vi "总磷氨氮插入数据.vi"(0 "database":string, 1 "data":T2 {"单位" items=["ug/L", "mg/L", "ppm", "mg/m3", "cm", "ppb", "ug/m3", "%", "nmol/mol", "umol/mol", "MPN/L", "MPN/100ml", "ng/m3", "NTU", "无量纲", "ms/cm", "us/cm"]}, 3 "SN":string, 5 "table":string, 7 "测量模式":T1(ring)=enum."水样测试", 9 "数据标记表":string(combo)="N", 11 "error in (no error)":errorcluster) -> (15 "error out":errorcluster)   [LabVIEW 2016, in "database.lvlib"]
uses:
  database.lvlib
  <vilib>/Utility/sysdir.llb/System Directory Type.ctl
  <vilib>/addons/database/Connection.llb/DB Tools Open Connec (String).vi
  <vilib>/addons/database/Connection.llb/Conn Execute.vi
  <vilib>/addons/database/Recordset.llb/Rec Fetch Recordset Data (R).vi
  <vilib>/addons/database/Recordset.llb/Rec Destroy - Connection.vi
  <vilib>/addons/database/NI_Database_API.lvlib
panel:
  out "为空？":bool
  out "recordset data":variant[][](array[variant])
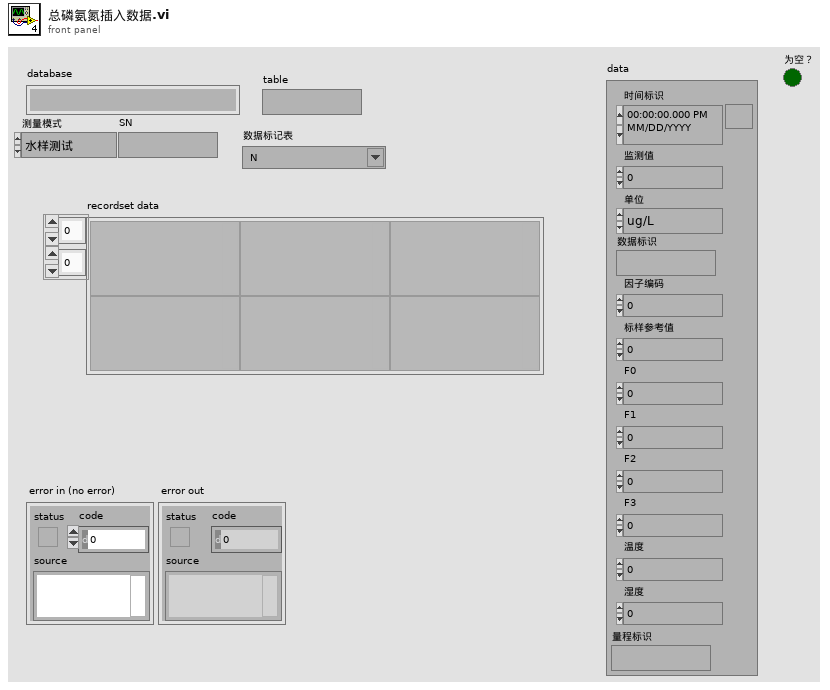
[diagram p1: front panel]
types:
  T1 = enum16{"维护数据", "水样测试", "标样核查", "零点核查", "跨度核查", "空白测试", "平行样测试", "加标回收", "空白校准", "标样校准", "初始化（清洗）"}
  T2 = cluster{"时间标识":timestamp, "监测值":sgl, "单位":u16, "数据标识":string, "因子编码":u32, "标样参考值":sgl, "F0":sgl, "F1":sgl, "F2":sgl, "F3":sgl, "温度":sgl, "湿度":sgl, "量程标识":string}
  T3 = typedef "System Directory Type.ctl" = i32
  T4 = typedef "NI_Database_API.lvlib/Conn ObjectReference.ctl" = refnum<k1>
  T5 = typedef "NI_Database_API.lvlib/Rec ObjectReference.ctl" = refnum<k1>
  T6 = cluster{"时间标识":timestamp, "测量模式":string, "数据类型":string, "监测值":sgl, "单位":string, "数据标识":string, "因子编码":string, "标样参考值":sgl, "F0":sgl, "F1":sgl, "F2":sgl, "F3":sgl, "温度":sgl, "湿度":sgl, "量程标识":string, "SN":string}
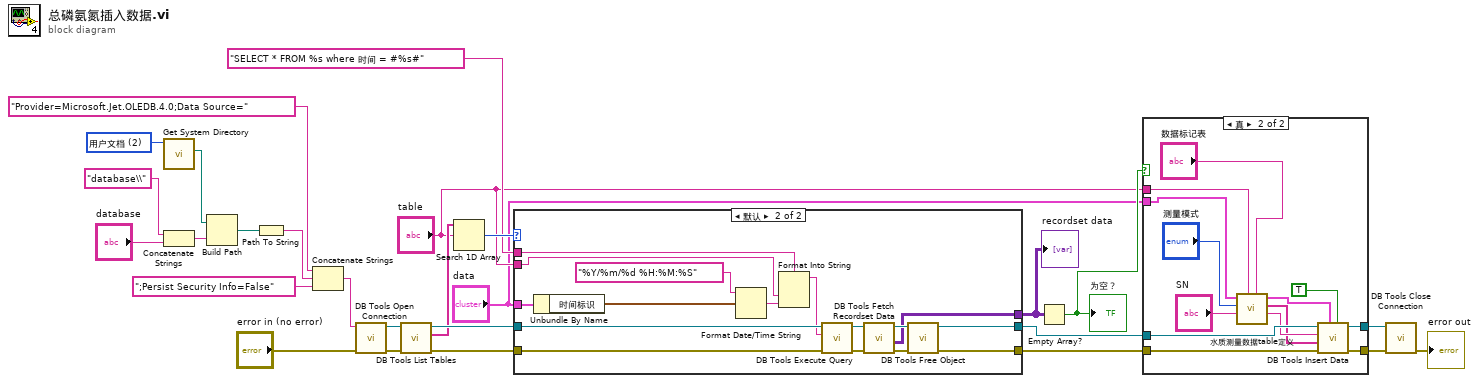
[diagram p0: block diagram]
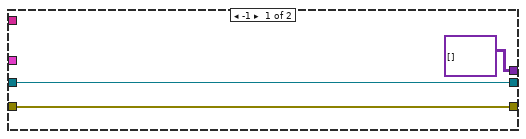
[diagram p3: hidden frame]
diagram:
  w26 = T3 2 items=["用户目录"=0, "用户桌面"=1, "用户文档"=2, "用户应用程序数据"=3, "用户设置"=4, "用户临时目录"=5, "公共文档"=6, "公共应用程序数据"=7, "公共设置"=8, "公共缓存"=13, "系统核心库"=9, "系统安装库"=10, "应用程序文件"=11, "启动盘根目录"=12] ("system directory type")
  n1 = call <vilib>:"Get System Directory.vi"("system directory type"=w26) -> ("system directory"=w24:path)  [unwired: 10 in]
  n2 = Concatenate Strings("database\\" ("condition"), "database") -> (w18:string)
  n3 = Build Path(base path=w24, name or relative path=w18) -> (appended path=w23:path)
  n4 = Path To String(path=w23) -> (string=w22:string)
  n5 = Concatenate Strings("Provider=Microsoft.Jet.OLEDB.4.0;Data Source=" ("condition"), w22, ";Persist Security Info=False" ("condition")) -> (w20:string)
  n6 = call-poly <vilib>:"DB Tools Open Connection.vi"("error in (no error)"="error in (no error)", "connection information"=w20) -> ("error out"=w15:errorcluster, "connection reference"=w16:T4)  [unwired: 6 in]
  n7 = call <vilib>:"DB Tools List Tables.vi"("error in (no error)"=w15, "connection reference"=w16) -> ("error out"=w13:errorcluster, "tables"=w12:string[], "connection reference out"=w14:T4)  [unwired: 3 in]
  n8 = Search 1D Array(1D array=w12, element="table") -> (index of element=w11:i32)  [unwired: 1 in]
  n9 = case shown="默认" w11 {
    tunnel: [variant[][] [] ("recordset data") w42] -> w17
    tunnel: [w30 w41] -> w4
    tunnel: [w29 w40] -> w5
    tunnel: w14 -> [w30 w39]
    tunnel: w13 -> [w29 w38]
    tunnel: "table" -> [_ w37]
    tunnel: "SELECT * FROM %s where 时间 = #%s#" ("格式字符串") -> [_ w36]
    tunnel: "data" -> [_ w31]
    frame -1 {
    }
    frame Default {
      n10 = Unbundle By Name(w31) -> ("时间标识"=w34:timestamp)
      n11 = Format Date/Time String(time format string (%c)="%Y/%m/%d %H:%M:%S" ("时间格式字符串(%c)"), seconds (now)=w34) -> (date/time string=w32:string)  [unwired: 1 in]
      n12 = Format Into String(format string=w36, w37, w32) -> (resulting string=w35:string)  [unwired: 2 in, 1 out]
      n13 = call-poly <vilib>:"DB Tools Execute Query.vi"("error in (no error)"=w38, "SQL query"=w35, "connection reference"=w39) -> ("error out"=w43:errorcluster, "recordset reference"=w46:T5)  [unwired: 5 in]
      n14 = call-poly <vilib>:"DB Tools Fetch Recordset Data.vi"("error in (no error)"=w43, "recordset reference"=w46) -> ("error out"=w44:errorcluster, "recordset data"=w42:variant[][], "recordset reference out"=w45:T5)  [unwired: 3 in]
      n15 = call-poly <vilib>:"DB Tools Free Object.vi"("error in (no error)"=w44, "recordset reference"=w45) -> ("error out"=w40:errorcluster, "connection reference"=w41:T4)  [unwired: 8 in]
    }
  }
  "recordset data" <- w17
  n16 = Empty Array?(array=w17) -> (empty?=w8:bool)
  "为空？" <- w8
  n17 = case shown="真" w8 {
    tunnel: "table" -> [_ w61]
    tunnel: "data" -> [_ w60]
    tunnel: w5 -> [w47 w58]
    tunnel: w4 -> [w48 w57]
    tunnel: [w48 w52] -> w3
    tunnel: [w47 w51] -> w2
    frame False {
    }
    frame True {
      n18 = call "水质测量数据table定义.vi"("数据标记表"="数据标记表", "table 输入"=w61, "SN"="SN", "测量模式"="测量模式", "data"=w60) -> ("table 输出"=w54:string, "columns"=w53:string[], "data输出"=w56:T6)  [unwired: 4 in]
      n19 = call <vilib>:"DB Tools Insert Data.vi"("create table? (F)"=TRUE, "data"=w56, "error in (no error)"=w58, "columns"=w53, "table"=w54, "connection reference"=w57) -> ("error out"=w51:errorcluster, "connection reference out"=w52:T4)  [unwired: 4 in]
    }
  }
  n20 = call <vilib>:"DB Tools Close Connection.vi"("error in (no error)"=w2, "connection reference"=w3) -> ("error out"=→"error out":errorcluster)  [unwired: 5 in]
